vi "登录界面示例.vi"() -> ()   [LabVIEW 2014]
panel:
  in  "显示密码":bool
  out "loading":string
  out "Status":string
  out "进度条":i32(slide) scale=0.0..100.0
  in  "取消按钮":bool
  in  "登录按钮":bool
  in  "密码":string
  in  "用户":string
  # "选中前面板垂直滚动条，右键属性--背景，可设置前面板背景图像"
  # "登录界面示例XXX系统"
  # "此处为用户名及密码；界面自行设计布局"
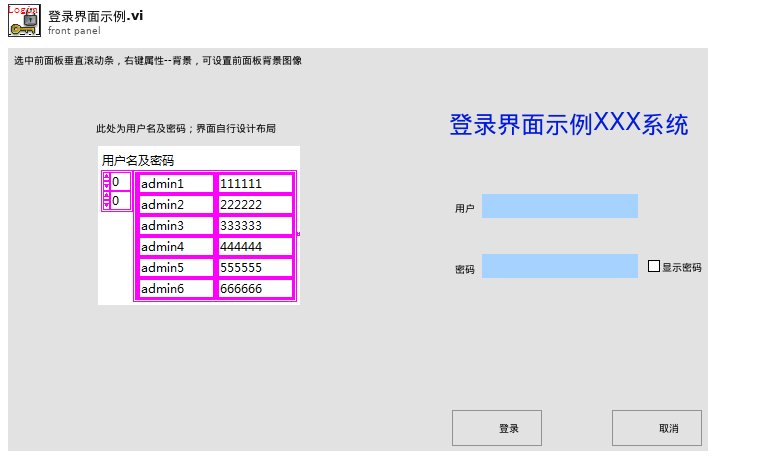
[diagram p1: front panel]
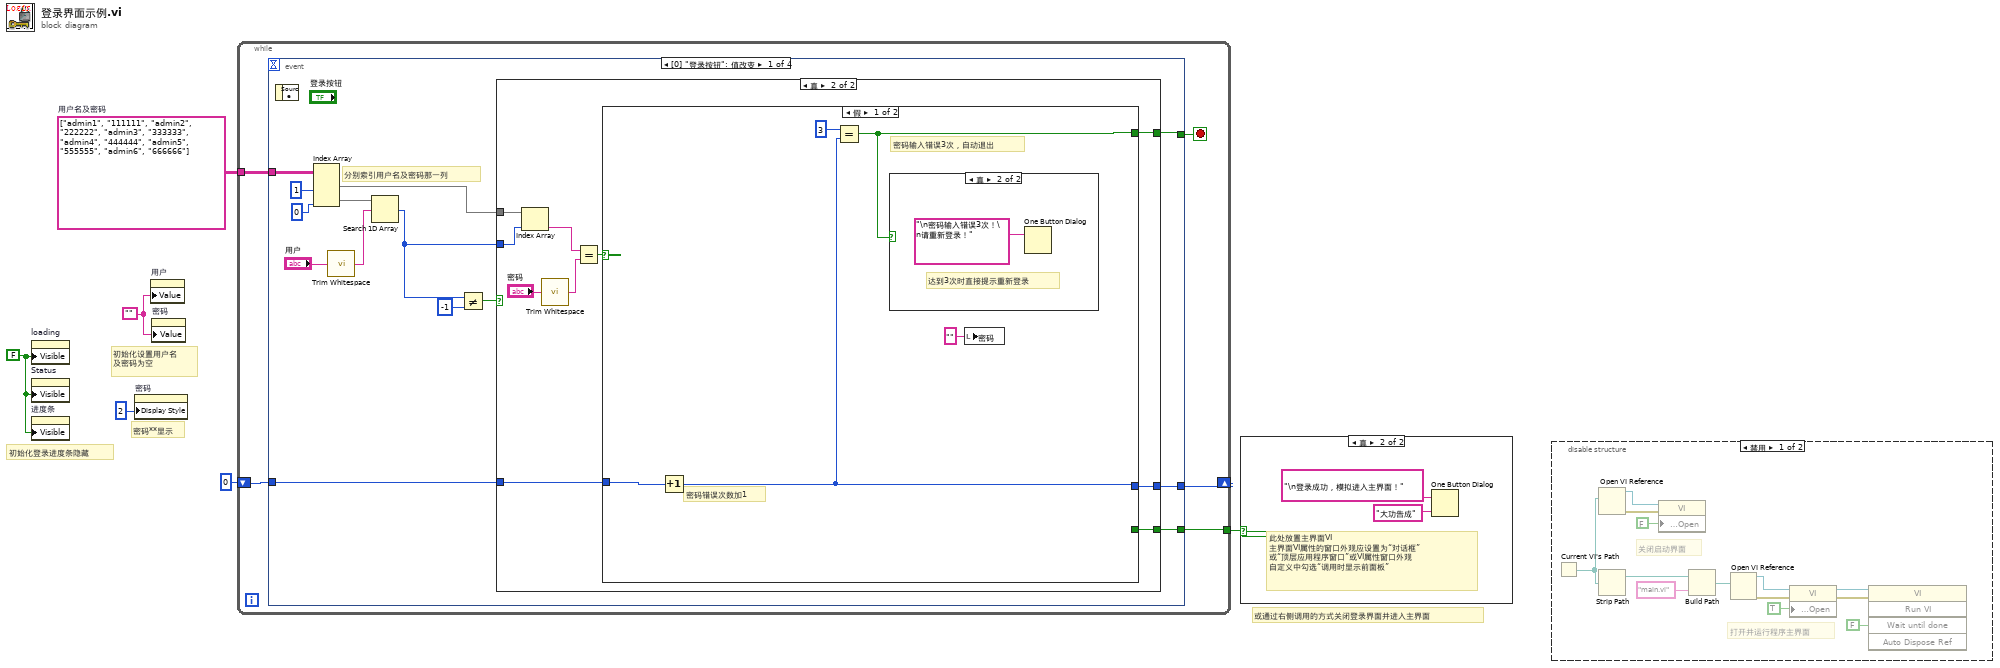
[diagram p0: block diagram]
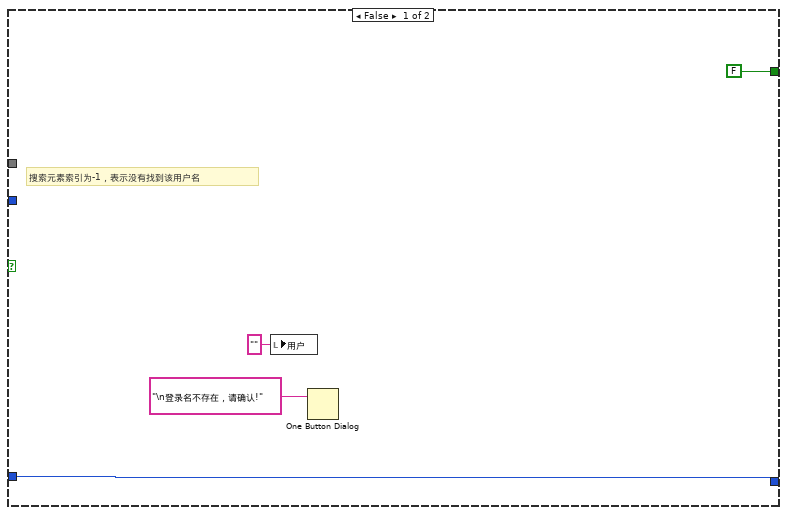
[diagram p4: hidden frame]
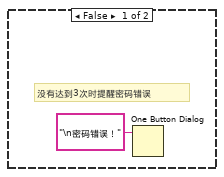
[diagram p5: hidden frame]
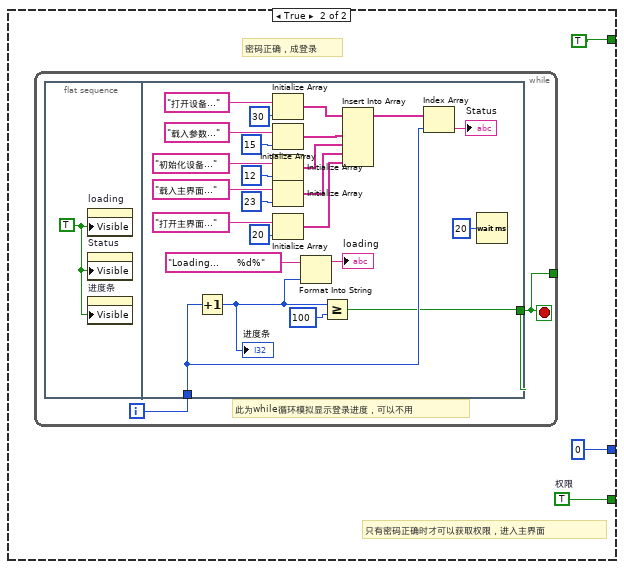
[diagram p6: hidden frame]
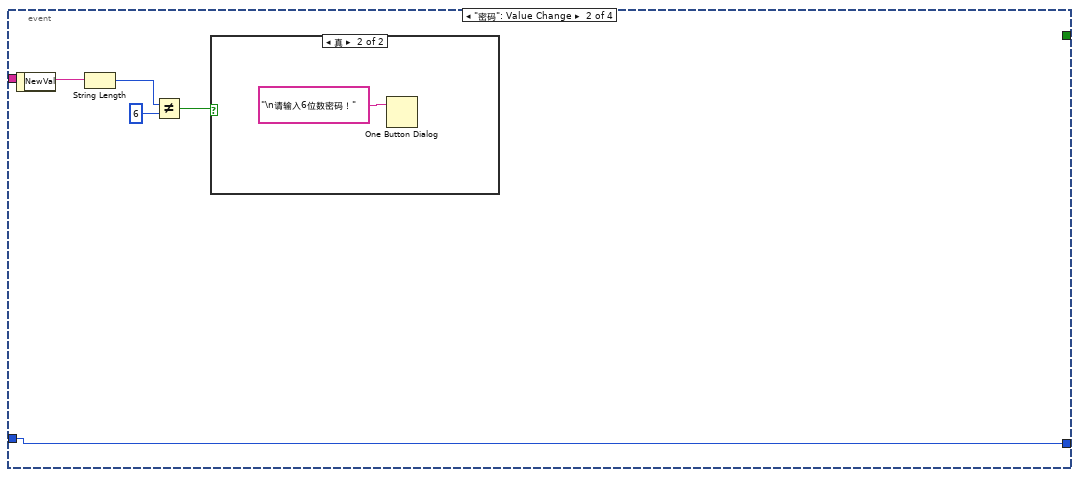
[diagram p7: hidden frame]
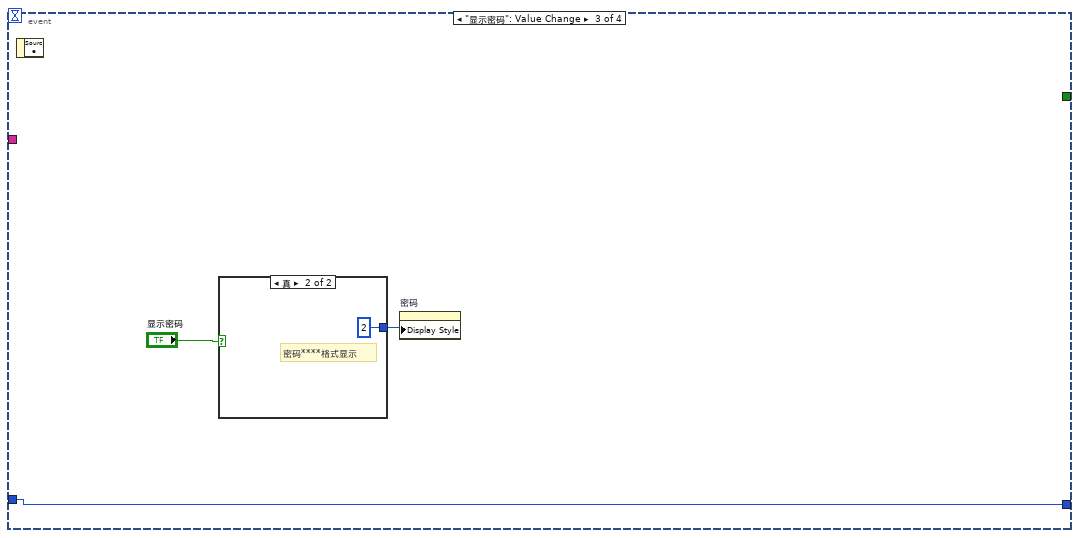
[diagram p9: hidden frame]
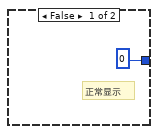
[diagram p10: hidden frame]
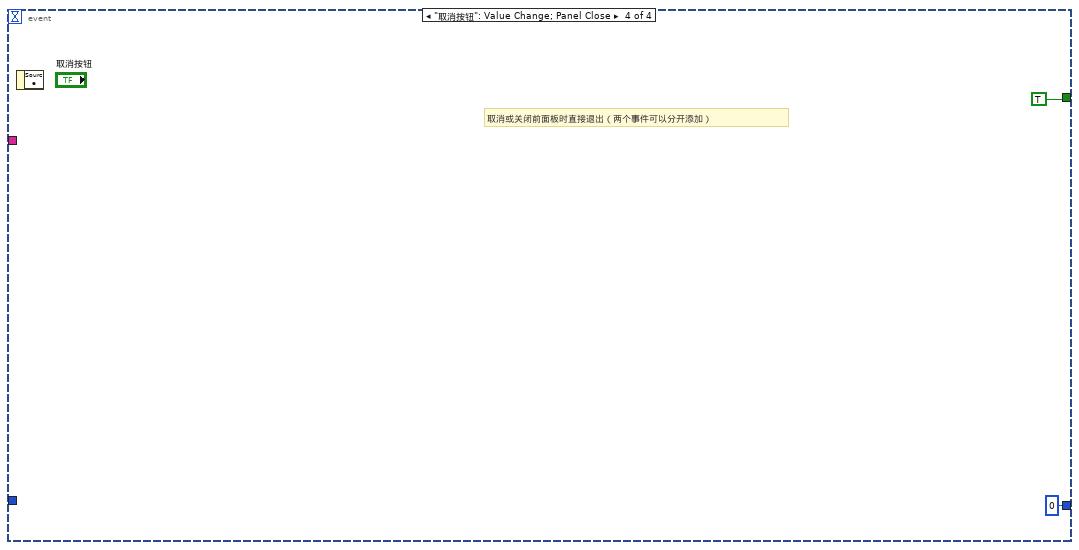
[diagram p11: hidden frame]
diagram:
  w3 = FALSE ("可见")
  w5 = string[][] [["admin1", "111111"], ["admin2", "222222"], ["admin3", "333333"], ["admin4", "444444"], ["admin5", "555555"], ["admin6", "666666"]]  # 用户名及密码
  w6 = ""
  # "或通过右侧调用的方式关闭登录界面并进入主界面"
  # "密码**显示"
  # "初始化登录进度条隐藏"
  # "初始化设置用户名\n及密码为空"
  n1 = property on="loading" class="Str"("Visible"=w3) -> ()  [unwired: 2 in, 2 out]
  n2 = property on="Status" class="Str"("Visible"=w3) -> ()  [unwired: 2 in, 2 out]
  n3 = property on="进度条" class="Slide (严格)"("Visible"=w3) -> ()  [unwired: 2 in, 2 out]
  n4 = property on="密码" class="Str"("Display Style"=u32 2 ("显示样式")) -> ()  [unwired: 2 in, 2 out]
  n5 = property on="用户" class="Str"("Value"=w6) -> ()  [unwired: 2 in, 2 out]
  n6 = property on="密码" class="Str"("Value"=w6) -> ()  [unwired: 2 in, 2 out]
  n7 = while {
    tunnel: w5 -> [w11]
    shift-right: [w8] -> _
    shift-left: 0 -> [w9]
    tunnel: [w7] -> w2
    stop <- w10 stop-if-true
    n8 = event shown="[0] \"登录按钮\": 值改变" {
      selector: _ -> [_ _ _ _]
      dyn-events: _ -> [_ _ _ _]
      timeout: _ -> [_ _ _ _]
      tunnel: w11 -> [w25 _ _ _]
      tunnel: [w13 _ _ TRUE] -> w10
      tunnel: w9 -> [w15 w77 w83 _]
      tunnel: [w14 w77 w83 0] -> w8
      tunnel: [w12 _ _ _] -> w7
      event "登录按钮": Value Change {
        # "分别索引用户名及密码那一列"
        n9 = event-data() -> ()  [unwired: 1 in, 1 out]
        n10 = Index Array(array=w25, index (col) #1=1 ("索引 (行)"), index (col) #2=0 ("禁用的索引 (列)")) -> (element #1=w17:string[], element #2=w22:string[])  [unwired: 2 in]
        n11 = call <vilib>:"Trim Whitespace.vi"("string"="用户") -> ("trimmed string"=w20:string)  [unwired: 1 in]
        n12 = Search 1D Array(1D array=w22, element=w20) -> (index of element=w16:i32)  [unwired: 1 in]
        n13 = Not Equal?(x=w16, y=-1) -> (x != y?=w18:bool)
        n14 = case shown="真" w18 {
          tunnel: w17 -> [_ w39]
          tunnel: w16 -> [_ w34]
          tunnel: [w27 w33] -> w14
          tunnel: w15 -> [w27 w32]
          tunnel: [FALSE w31] -> w13
          tunnel: [_ w30] -> w12
          frame False {
            # "搜索元素索引为-1，表示没有找到该用户名"
            n15 = local write "用户"("" ("用户")) -> ()
            n16 = One Button Dialog(message="\n登录名不存在，请确认!") -> ()  [unwired: 1 in, 1 out]
          }
          frame True {
            n17 = Index Array(array=w39, index=w34) -> (element=w36:string)
            n18 = call <vilib>:"Trim Whitespace.vi"("string"="密码") -> ("trimmed string"=w37:string)  [unwired: 1 in]
            n19 = Equal?(x=w36, y=w37) -> (x = y?=w35:bool)
            n20 = case shown="假" w35 {
              tunnel: [w43 0] -> w33
              tunnel: w32 -> [w44 _]
              tunnel: [w41 TRUE] -> w31
              tunnel: [_ w47] -> w30
              frame False {
                # "密码输入错误3次，自动退出"
                # "密码错误次数加1"
                n21 = Increment(x=w44) -> (x+1=w43:i32)
                n22 = Equal?(x=3, y=w43) -> (x = y?=w41:bool)
                n23 = case shown="真" w41 {
                  frame False {
                    # "没有达到3次时提醒密码错误"
                    n24 = One Button Dialog(message="\n密码错误！") -> ()  [unwired: 1 in, 1 out]
                  }
                  frame True {
                    # "达到3次时直接提示重新登录"
                    n25 = One Button Dialog(message="\n密码输入错误3次！\n请重新登录！") -> ()  [unwired: 1 in, 1 out]
                  }
                }
                n26 = local write "密码"("" ("密码")) -> ()
              }
              frame True {
                w47 = TRUE  # 权限
                # "只有密码正确时才可以获取权限，进入主界面"
                # "密码正确，成登录"
                n27 = while {
                  tunnel: [w50] -> _
                  i -> [w51]
                  stop <- w50 stop-if-true
                  # "此为while循环模拟显示登录进度，可以不用"
                  n28 = flat-sequence {
                    tunnel: w51 -> [w54]
                    tunnel: [w53] -> w50
                    frame #0 {
                      w52 = TRUE ("可见")
                      n29 = property on="loading" class="Str"("Visible"=w52) -> ()  [unwired: 2 in, 2 out]
                      n30 = property on="Status" class="Str"("Visible"=w52) -> ()  [unwired: 2 in, 2 out]
                      n31 = property on="进度条" class="Slide (严格)"("Visible"=w52) -> ()  [unwired: 2 in, 2 out]
                    }
                    frame #1 {
                      n32 = Increment(x=w54) -> (x+1=w55:i32)
                      "进度条" <- w55
                      n33 = Initialize Array("打开设备...", 30 ("维数大小")) -> (w61:string[])
                      n34 = Initialize Array("载入参数...", 15 ("维数大小")) -> (w60:string[])
                      n35 = Initialize Array("初始化设备...", 12 ("维数大小")) -> (w59:string[])
                      n36 = Initialize Array("载入主界面...", 23 ("维数大小")) -> (w58:string[])
                      n37 = Initialize Array("打开主界面...", 20 ("维数大小")) -> (w57:string[])
                      n38 = Format Into String(format string="Loading...      %d%", w55) -> (resulting string=→"loading":string)  [unwired: 2 in, 1 out]
                      n39 = Greater Or Equal?(x=w55, y=100) -> (x >= y?=w53:bool)
                      n40 = Insert Into Array(array=w61, new element #1=w60, new element #2=w59, new element #3=w58, new element #4=w57) -> (w56:string[])  [unwired: 1 in]
                      n41 = Index Array(array=w56, index=w54) -> (element=→"Status":string)
                      n42 = Wait (ms)(milliseconds to wait=u32 20) -> ()  [unwired: 1 out]
                    }
                  }
                }
              }
            }
          }
        }
      }
      event "密码": Value Change {
        n43 = event-data() -> ("NewVal"=w81:string)  [unwired: 1 in]
        n44 = String Length(string=w81) -> (length=w80:i32)
        n45 = Not Equal?(x=w80, y=6) -> (x != y?=w78:bool)
        n46 = case shown="真" w78 {
          frame False {
          }
          frame True {
            n47 = One Button Dialog(message="\n请输入6位数密码！") -> ()  [unwired: 1 in, 1 out]
          }
        }
      }
      event "显示密码": Value Change {
        n48 = event-data() -> ()  [unwired: 1 in, 1 out]
        n49 = case shown="真" "显示密码" {
          tunnel: [u32 0 ("显示样式") u32 2 ("显示样式")] -> w84
          frame False {
            # "正常显示"
          }
          frame True {
            # "密码****格式显示"
          }
        }
        n50 = property on="密码" class="Str"("Display Style"=w84) -> ()  [unwired: 2 in, 2 out]
      }
      event "取消按钮": Value Change; Panel Close {
        # "取消或关闭前面板时直接退出（两个事件可以分开添加）"
        n51 = event-data() -> ()  [unwired: 1 in, 1 out]
      }
    }
  }
  n52 = case shown="真" w2 {
    frame False {
      # "没有获取权限，不进入主界面"
    }
    frame True {
      # "此处放置主界面VI\n主界面VI属性的窗口外观应设置为“对话框”\n或“顶层应用程序窗口”或VI属性窗口外观\n自定义中勾选“调用时显示前面板”"
      n53 = One Button Dialog(message="\n登录成功，模拟进入主界面！", button name ("OK")="大功告成" ("按钮名称（“确定”）")) -> ()  [unwired: 1 out]
    }
  }
  n54 = disable-structure shown="禁用" {
    frame Disabled {
      # "打开并运行程序主界面"
      # "关闭启动界面"
      n55 = Current VI's Path() -> (path=w92:path)
      n56 = Open VI Reference(vi path=w92) -> (vi reference=w103:refnum<vi>, error out=w101:errorcluster)  [unwired: 2 in, 3 out]
      n57 = Strip Path(path=w92) -> (stripped path=w93:path)  [unwired: 1 out]
      n58 = property on="Property Node" class="VI"(reference=w103, error in=w101, "Front Panel Window:Open"=FALSE) -> ()  [unwired: 2 out]
      n59 = Build Path(base path=w93, name or relative path="main.vi") -> (appended path=w94:path)
      n60 = Open VI Reference(vi path=w94) -> (vi reference=w95:refnum<vi>, error out=w96:errorcluster)  [unwired: 2 in, 3 out]
      n61 = property on="Property Node" class="VI"(reference=w95, error in=w96, "Front Panel Window:Open"=TRUE) -> (reference out=w98:refnum<vi>, error out=w99:errorcluster)
      n62 = invoke class="VI" method="Run VI"(reference=w98, error in=w99, "Wait until done"=FALSE) -> ()  [unwired: 2 in, 5 out]
    }
    frame Enabled {
    }
  }
